vi "Polar Deadband.vi"(8 "Value to Deadband (default of 0.1)":dbl, 10 "Y Axis":dbl, 11 "X Axis":dbl) -> (0 "Joystick Y Axis":dbl, 1 "Joystick X Axis":dbl, 2 "Joystick Magnitude":dbl, 3 "Joystick Degree":dbl)   [LabVIEW 2013]
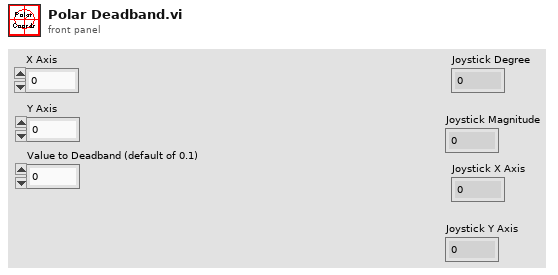
[diagram p1: front panel]
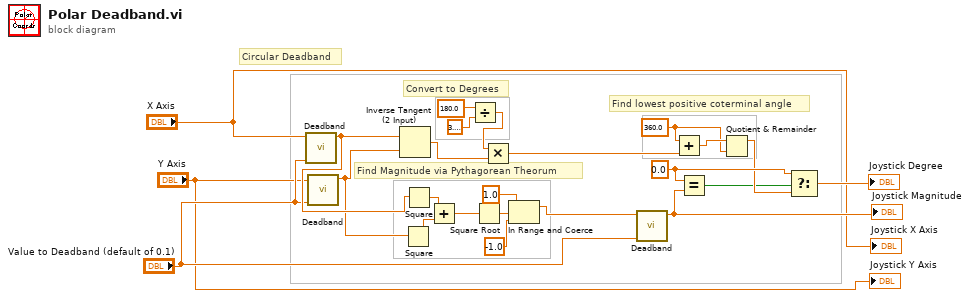
[diagram p0: block diagram]
diagram:
  w11 = 0.0 ("x")
  w12 = 360.0 ("x")
  # "Find lowest positive coterminal angle"
  # "Convert to Degrees"
  # "Find Magnitude via Pythagorean Theorum"
  # "Circular Deadband"
  n1 = call "Deadband.vi"("Value to Deadband (default of 0.1)"="Value to Deadband (default of 0.1)", "Value"="X Axis") -> ("Deadbanded Value"=w8:dbl)  [unwired: 9 in]
  n2 = call "Deadband.vi"("Value to Deadband (default of 0.1)"="Value to Deadband (default of 0.1)", "Value"="Y Axis") -> ("Deadbanded Value"=w7:dbl)  [unwired: 9 in]
  n3 = Inverse Tangent (2 Input)(1:w7, 2:w8) -> (0:w14:dbl)
  n4 = Square(x=w7) -> (x^2=w24:dbl)
  n5 = Square(x=w8) -> (x^2=w23:dbl)
  n6 = Add(x=w23, y=w24) -> (x+y=w22:dbl)
  n7 = Divide(x=180.0, y=3.141592653589793) -> (x/y=w15:dbl)
  n8 = Square Root(x=w22) -> (sqrt(x)=w21:dbl)
  n9 = Multiply(x=w15, y=w14) -> (x*y=w1:dbl)
  n10 = In Range and Coerce(upper limit=1.0, x=w21, lower limit=-1.0) -> (coerced(x)=w18:dbl)  [unwired: 1 out]
  n11 = call "Deadband.vi"("Value to Deadband (default of 0.1)"="Value to Deadband (default of 0.1)", "Value"=w18) -> ("Deadbanded Value"=w4:dbl)  [unwired: 9 in]
  "Joystick Magnitude" <- w4
  n12 = Add(x=w12, y=w1) -> (x+y=w13:dbl)
  n13 = Equal?(x=w11, y=w4) -> (x = y?=w9:bool)
  n14 = Quotient & Remainder(x=w13, y=w12) -> (x-y*floor(x/y)=w10:dbl)  [unwired: 1 out]
  n15 = Select(t=w11, s=w9, f=w10) -> (s? t:f=→"Joystick Degree":dbl)
  "Joystick Y Axis" <- "Y Axis"
  "Joystick X Axis" <- "X Axis"
